vi "Joystick Begin.vi"(9 "error in (no error)":errorcluster) -> (0 "error out":errorcluster)   [LabVIEW 2013]
uses:
  <vilib>/Rock Robotics/WPI/Joystick/WPI_JoystickDeviceEnum.ctl
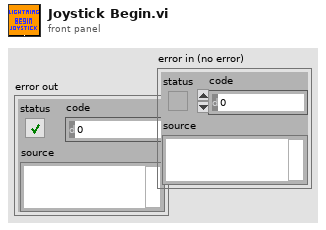
[diagram p1: front panel]
types:
  T1 = typedef "WPI_JoystickDeviceEnum.ctl" = enum16{"USB 1", "USB 2", "USB 3", "USB 4", "Kinect 1", "Kinect 2"}
  T2 = typedef "WPI_JoystickDevRef.ctl" = cluster{"Device":T1}
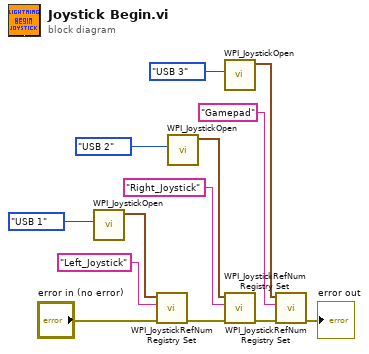
[diagram p0: block diagram]
diagram:
  n1 = call <vilib>:"WPI_JoystickOpen.vi"("JoystickDevice"=WPI_JoystickDeviceEnum."USB 1") -> ("JoystickDevRef"=w3:T2)  [unwired: 10 in]
  n2 = call <vilib>:"WPI_JoystickRefNum Registry Set.vi"("error in (no error)"="error in (no error)", "refnum name"="Left_Joystick", "JoystickDevRef"=w3) -> ("error out"=w8:errorcluster)  [unwired: 7 in, 1 out]
  n3 = call <vilib>:"WPI_JoystickOpen.vi"("JoystickDevice"=WPI_JoystickDeviceEnum."USB 2") -> ("JoystickDevRef"=w6:T2)  [unwired: 10 in]
  n4 = call <vilib>:"WPI_JoystickOpen.vi"("JoystickDevice"=WPI_JoystickDeviceEnum."USB 3") -> ("JoystickDevRef"=w10:T2)  [unwired: 10 in]
  n5 = call <vilib>:"WPI_JoystickRefNum Registry Set.vi"("error in (no error)"=w8, "refnum name"="Right_Joystick", "JoystickDevRef"=w6) -> ("error out"=w12:errorcluster)  [unwired: 7 in, 1 out]
  n6 = call <vilib>:"WPI_JoystickRefNum Registry Set.vi"("error in (no error)"=w12, "refnum name"="Gamepad", "JoystickDevRef"=w10) -> ("error out"=→"error out":errorcluster)  [unwired: 7 in, 1 out]
